vi "Create TDMS map file.vi"(4 "Sample name":string, 6 "Description":string, 7 "Folder path":path, 8 "Operator":string, 9 "Sample holder":T2, 10 "Map parameters":T3={"B_start[T]"=0.0, "B_End[T]"=0.0, "B_rate [mT/s]"=0.0, "F_start[GHz]"=0.0, "F_end[GHz]"=0.0, "Sampling rate"=0, "Tmp [K]"=295.0, "Wait[min]"=0.0, "Points"=0, "Display signal"=enum."Phi", "Signal treat"=enum."None", "Sweep [s]"=2.0} {"Sampling rate" items=["117 ks/S"=9, "58.6 kS/s"=10, "29.3 kS/s"=11, "14.6 kS/s"=12, "7.32 kS/s"=13, "3.66 kS/s"=14, "1.83 kS/s"=15]}, 11 "ACQ parameters":T1 {"Enable output" items=["Disable", "Enable"]; "Amp_Mod [mV]" min=0.0 max=10000.0; "F_Mod [kHz]" min=0.1 max=100.0; "Filter order" min=1.0 max=9.0 step=1.0; "Time constant [ms]" min=0.0 max=1000.0}) -> (0 "error out":errorcluster, 3 "tdms map file out":refnum<k34>)   [LabVIEW 2024]
uses:
  Datatypes/Map parameters.ctl
  Subsystem modules/Lock-in module/ctl/OSC sampling rate.ctl
  Datatypes/SampleHolders.ctl
  Subsystem modules/Lock-in module/ctl/MFLI parameters.ctl
  <vilib>/Utility/sysdir.llb/System Directory Type.ctl
  Subsystem modules/Lock-in module/Lock-in module.lvlib
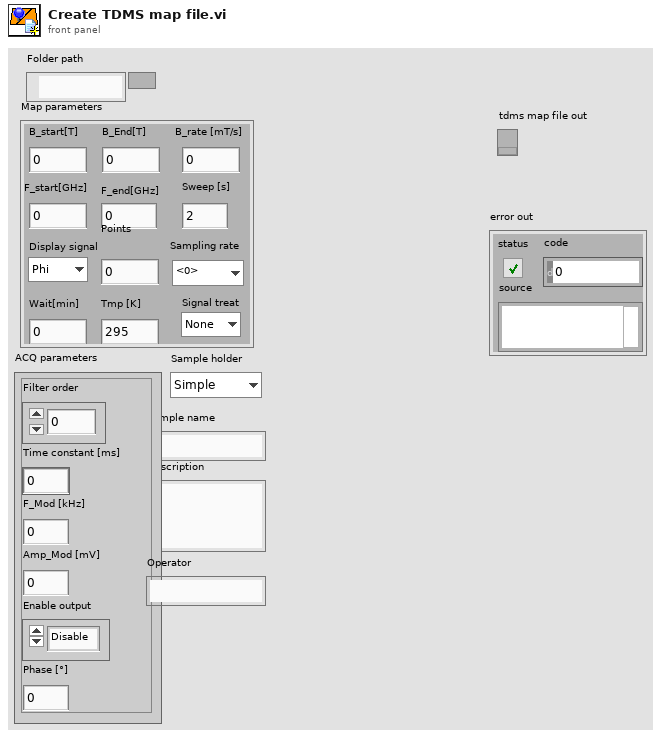
[diagram p1: front panel]
types:
  T1 = typedef "Lock-in module.lvlib/MFLI parameters.ctl" = cluster{"Filter order":dbl, "Time constant [ms]":dbl, "F_Mod [kHz]":dbl, "Amp_Mod [mV]":dbl, "Enable output":u16, "Phase [°]":dbl}
  T2 = typedef "SampleHolders.ctl" = enum16{"Simple", "Carousel", "Chip", "Rotator", "Liquid"}
  T3 = typedef "Map parameters.ctl" = cluster{"B_start[T]":dbl, "B_End[T]":dbl, "B_rate [mT/s]":dbl, "F_start[GHz]":dbl, "F_end[GHz]":dbl, "Sampling rate":T4, "Tmp [K]":dbl, "Wait[min]":dbl, "Points":u32, "Display signal":enum16{"X", "Y", "R", "Phi"}, "Signal treat":enum16{"None", "Unity norm", "Mean norm", "Standardization"}, "Sweep [s]":dbl}
  T4 = typedef "OSC sampling rate.ctl" = u16
  T5 = typedef "System Directory Type.ctl" = i32
  T6 = enum16{"open", "open or create", "create or replace", "create", "open (read-only)"}
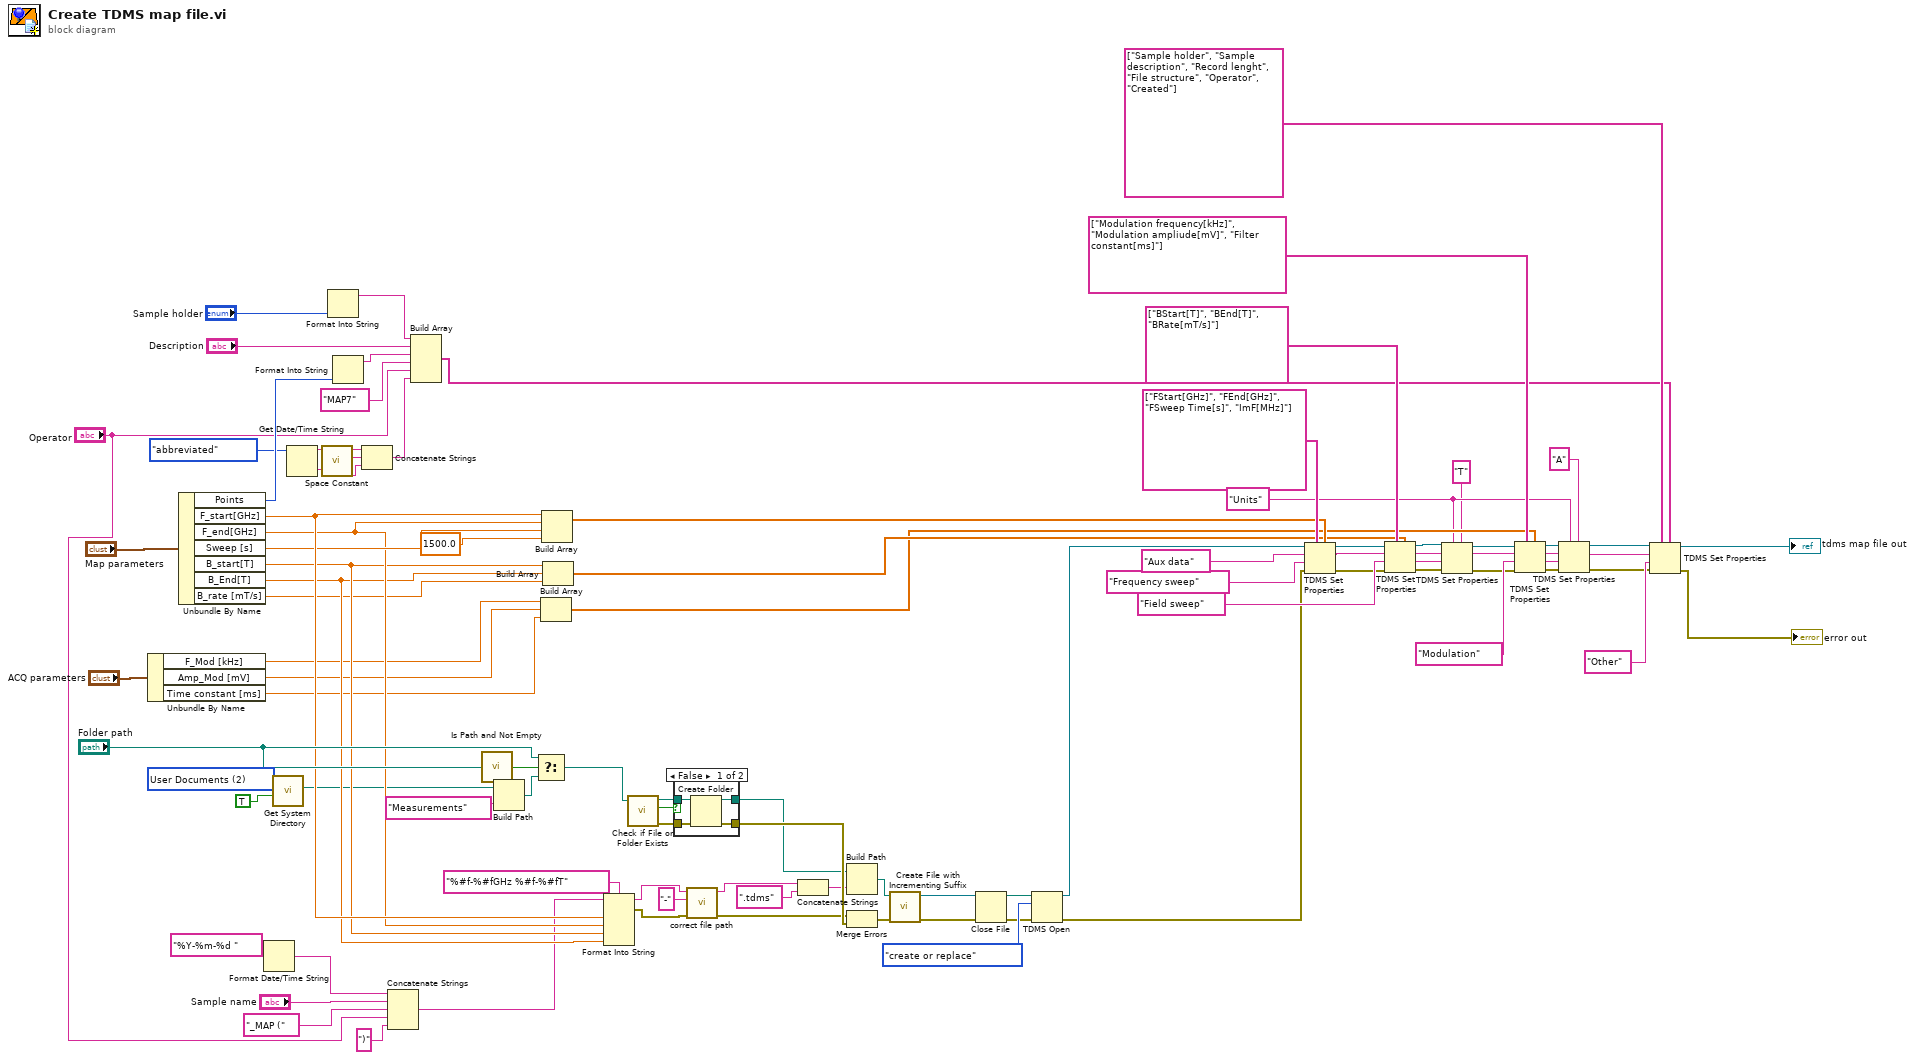
[diagram p0: block diagram]
diagram:
  w12 = T5 2 items=["User Home"=0, "User Desktop"=1, "User Documents"=2, "User Application Data"=3, "User Preferences"=4, "User Temporary"=5, "Public Documents"=6, "Public Application Data"=7, "Public Preferences"=8, "Public Cache"=13, "System Core Libraries"=9, "System Installed Libraries"=10, "Application Files"=11, "Boot Volume Root"=12] ("system directory type")
  w18 = "Units" ("property names")
  n1 = Unbundle By Name("ACQ parameters") -> ("F_Mod [kHz]"=w46:dbl, "Amp_Mod [mV]"=w45:dbl, "Time constant [ms]"=w44:dbl)
  n2 = Unbundle By Name("Map parameters") -> ("Points"=w34:u32, "F_start[GHz]"=w67:dbl, "F_end[GHz]"=w65:dbl, "Sweep [s]"=w66:dbl, "B_start[T]"=w49:dbl, "B_End[T]"=w48:dbl, "B_rate [mT/s]"=w47:dbl)
  n3 = Format Date/Time String(time format string (%c)="%Y-%m-%d ") -> (date/time string=w8:string)  [unwired: 2 in]
  n4 = call <vilib>:"Get System Directory.vi"("create directory if not found? (F)"=TRUE, "system directory type"=w12) -> ("system directory"=w10:path)  [unwired: 9 in]
  n5 = Get Date/Time String(date format (0)=enum16{"short", "long", "abbreviated"}."abbreviated") -> (date string=w5:string, time string=w4:string)  [unwired: 2 in]
  n6 = call <vilib>:"Space Constant.vi"() -> ("String"=w3:string)
  n7 = Format Into String("Sample holder") -> (resulting string=w39:string)  [unwired: 3 in, 1 out]
  n8 = Format Into String(w34) -> (resulting string=w33:string)  [unwired: 3 in, 1 out]
  n9 = Concatenate Strings(w5, w3, w4) -> (w2:string)
  n10 = Concatenate Strings(w8, "Sample name", "_MAP (", "Operator", ")" ("string")) -> (w31:string)
  n11 = Build Array(w39, "Description", w33, "MAP7" ("element"), "Operator", w2) -> (w37:string[])
  n12 = call <vilib>:"Is Path and Not Empty.vi"("path"="Folder path") -> ("Is Path and Not Empty?"=w85:bool)  [unwired: 4 in]
  n13 = Build Path(base path=w10, name or relative path="Measurements") -> (appended path=w86:path)
  n14 = Select(t="Folder path", s=w85, f=w86) -> (s? t:f=w9:path)
  n15 = Build Array(w46, w45, w44) -> (w41:dbl[])
  n16 = Build Array(w67, w65, w66, 1500.0 ("input 4")) -> (w43:dbl[])
  n17 = Build Array(w49, w48, w47) -> (w42:dbl[])
  n18 = Format Into String(format string="%#f-%#fGHz %#f-%#fT", initial string=w31, w67, w65, w49, w48) -> (resulting string=w76:string, error out=w81:errorcluster)  [unwired: 1 in]
  n19 = call <vilib>:"Check if File or Folder Exists.vi"("path"=w9) -> ("error out"=w83:errorcluster, "file or folder exists?"=w82:bool, "dup path"=w84:path)  [unwired: 8 in]
  n20 = case shown="False" w82 {
    tunnel: w84 -> [w97 w101]
    tunnel: [w98 w100] -> w88
    tunnel: w83 -> [w99 w100]
    tunnel: [w96 w101] -> w87
    frame False {
      n21 = Create Folder(path (use dialog)=w97, error in=w99) -> (created path=w96:path, error out=w98:errorcluster)  [unwired: 1 in, 1 out]
    }
    frame True {
    }
  }
  n22 = call "correct file path.vi"("error in (no error)"=w81, "replacement (-)"="-" ("replacement"), "input path"=w76) -> ("error out"=w79:errorcluster, "corrected path"=w75:string)  [unwired: 7 in]
  n23 = Concatenate Strings(w75, ".tdms" ("string")) -> (w77:string)
  n24 = Build Path(base path=w87, name or relative path=w77) -> (appended path=w78:path)
  n25 = Merge Errors(w79, w88) -> (w80:errorcluster)
  n26 = call <vilib>:"Create File with Incrementing Suffix.vi"("error in (no error)"=w80, "file path"=w78) -> ("error out"=w71:errorcluster, "refnum out"=w72:refnum<file>)  [unwired: 7 in, 1 out]
  n27 = Close File(refnum=w72, error in=w71) -> (path=w69:path, error out=w70:errorcluster)
  n28 = TDMS Open(8:w70, 10:T6."create or replace" ("operation (0:open)"), 11:w69) -> (0:w51:errorcluster, 3:w52:refnum<k34>)  [unwired: 4 in]
  n29 = TDMS Set Properties(5:w43, 7:string[] ["FStart[GHz]", "FEnd[GHz]", "FSweep Time[s]", "ImF[MHz]"], 8:w51, 9:"Frequency sweep" ("channel name"), 10:"Aux data" ("group name"), 11:w52) -> (0:w57:errorcluster, 2:w55:string, 3:w53:refnum<k34>)  [unwired: 1 out]
  n30 = TDMS Set Properties(5:w42, 7:string[] ["BStart[T]", "BEnd[T]", "BRate[mT/s]"], 8:w57, 9:"Field sweep", 10:w55, 11:w53) -> (0:w22:errorcluster, 1:w21:string, 2:w20:string, 3:w19:refnum<k34>)
  n31 = TDMS Set Properties(5:"T", 7:w18, 8:w22, 9:w21, 10:w20, 11:w19) -> (0:w14:errorcluster, 2:w15:string, 3:w16:refnum<k34>)  [unwired: 1 out]
  n32 = TDMS Set Properties(5:w41, 7:string[] ["Modulation frequency[kHz]", "Modulation ampliude[mV]", "Filter constant[ms]"], 8:w14, 9:"Modulation" ("channel name"), 10:w15, 11:w16) -> (0:w29:errorcluster, 1:w25:string, 2:w26:string, 3:w54:refnum<k34>)
  n33 = TDMS Set Properties(5:"A", 7:w18, 8:w29, 9:w25, 10:w26, 11:w54) -> (0:w28:errorcluster, 2:w24:string, 3:w30:refnum<k34>)  [unwired: 1 out]
  n34 = TDMS Set Properties(5:w37, 7:string[] ["Sample holder", "Sample description", "Record lenght", "File structure", "Operator", "Created"], 8:w28, 9:"Other" ("channel name"), 10:w24, 11:w30) -> (0:→"error out":errorcluster, 3:→"tdms map file out":refnum<k34>)  [unwired: 2 out]
